vi "APTpiezoOpen.vi"(4 "error in (no error)":errorcluster) -> (0 "error out":errorcluster, 3 "reference out":refnum<k7>)   [LabVIEW 2013]
panel:
  in  "MG17Piezo":refnum<k7>(container)
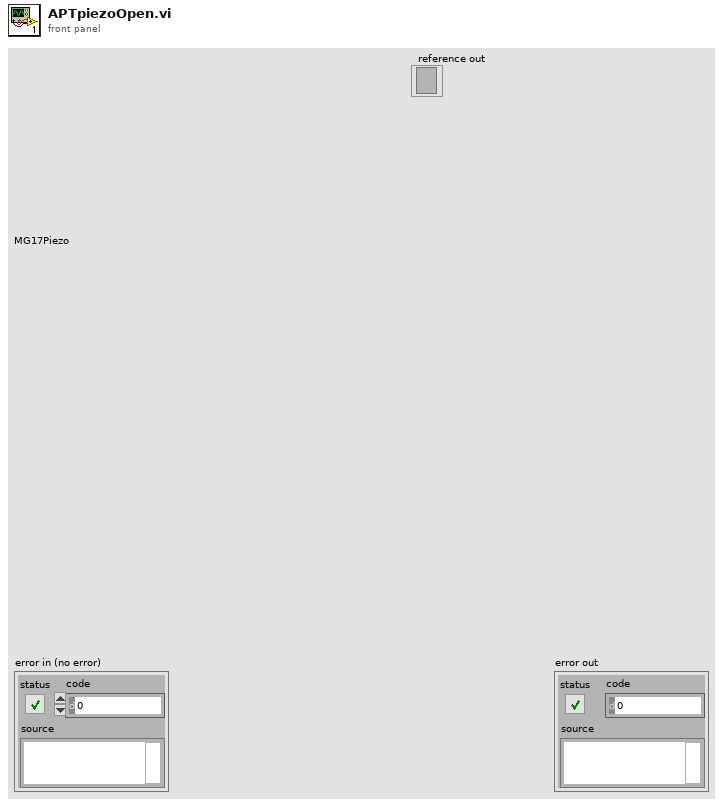
[diagram p1: front panel]
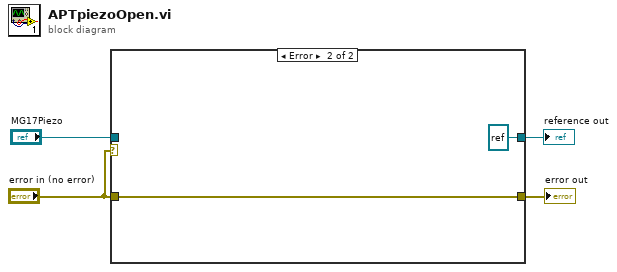
[diagram p0: block diagram]
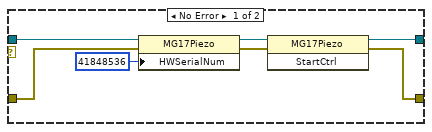
[diagram p2: hidden frame]
diagram:
  n1 = case shown="Error" "error in (no error)" {
    tunnel: "MG17Piezo" -> [w11 _]
    tunnel: "error in (no error)" -> [w7 w13]
    tunnel: [w6 w13] -> w3
    tunnel: [w5 refnum<k7> refnum ("MG17Piezo")] -> w2
    frame No Error {
      n2 = property class="MG17Piezo"(reference=w11, error in=w7, "HWSerialNum"=41848536) -> (reference out=w9:refnum<k7>, error out=w8:errorcluster)
      n3 = invoke class="MG17Piezo" method="StartCtrl"(reference=w9, error in=w8) -> (reference out=w5:refnum<k7>, error out=w6:errorcluster)  [unwired: 1 in, 1 out]
    }
    frame Error {
    }
  }
  "error out" <- w3
  "reference out" <- w2
